vi "Read Current (List Voltage Sweep).vi"(5 "Delay Time (0.5 S)":dbl=0.5, 7 "Sweep Points (5)":i32=5, 8 "error in (no error)":errorcluster, 9 "Sweep List (V)":dbl[](array[numeric]), 10 "Source Measure Unit Channel (0: Channel A)":i32(ring) items=["Channel A", "Channel B"], 11 "VISA resource name":refnum<visa-resource-name>) -> (0 "error out":errorcluster, 2 "Current (A)":dbl[](array[numeric]), 3 "VISA resource name out":refnum<visa-resource-name>)   [LabVIEW 2015, in "Keithley 2600 Series.lvlib"]
doc: "Performs a voltage list sweep with current measured at every point."
uses:
  Keithley 2600 Series.lvlib
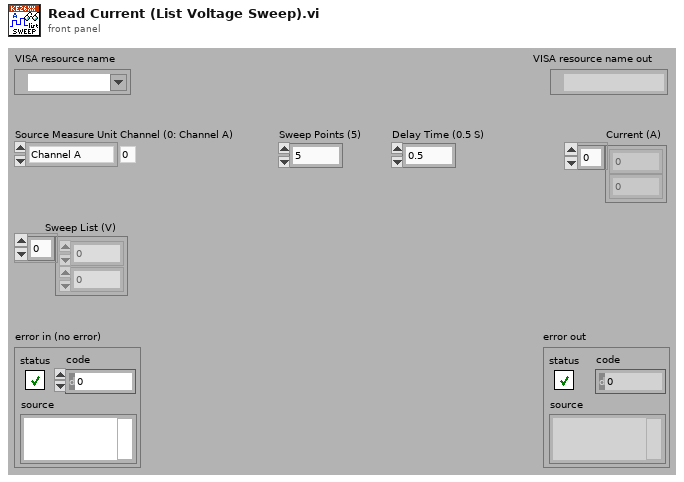
[diagram p1: front panel]
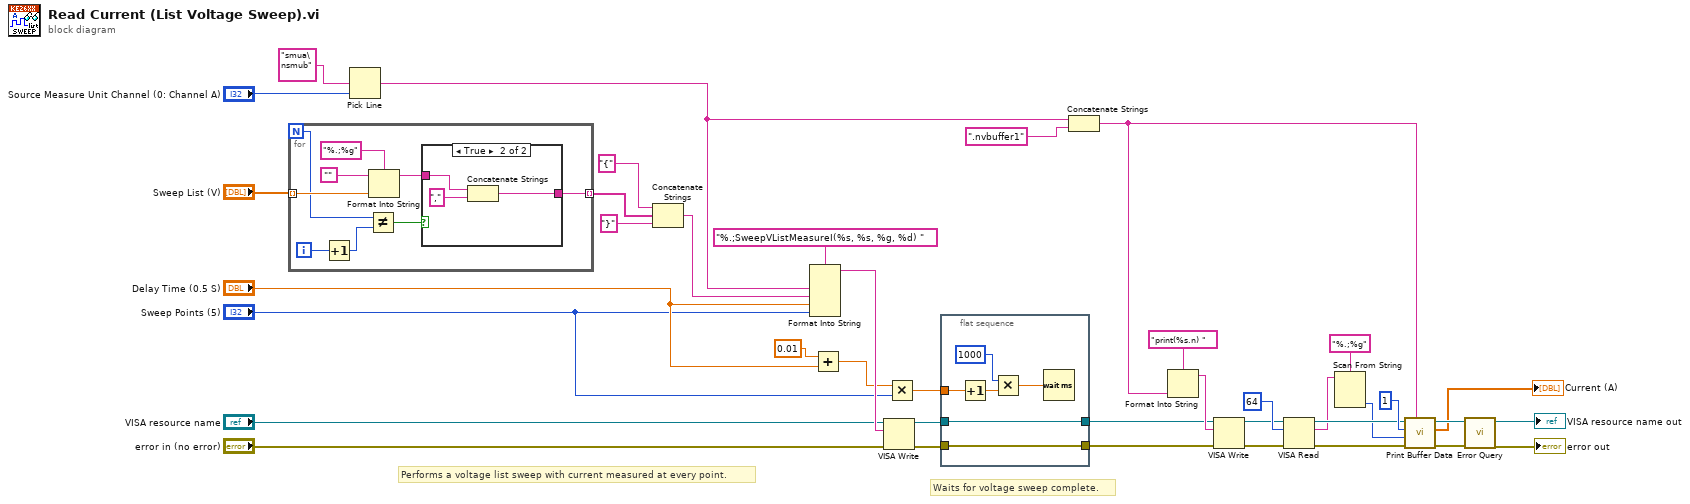
[diagram p0: block diagram]
diagram:
  # "Waits for voltage sweep complete."
  # "Performs a voltage list sweep with current measured at every point."
  n1 = for {
    N -> [w40]
    tunnel: "Sweep List (V)" -> [w48] mode=indexing
    tunnel: [w41] -> w31 mode=indexing
    i -> [w45]
    n2 = Increment(x=w45) -> (x+1=w44:i32)
    n3 = Not Equal?(x=w40, y=w44) -> (x != y?=w43:bool)
    n4 = Format Into String(format string="%.;%g", initial string="", w48) -> (resulting string=w42:string)  [unwired: 1 in, 1 out]
    n5 = case shown="True" w43 {
      tunnel: w42 -> [w49 w52]
      tunnel: [w49 w50] -> w41
      frame False {
      }
      frame True {
        n6 = Concatenate Strings(w52, ",") -> (w50:string)
      }
    }
  }
  n7 = Pick Line(multi-line string="smua\nsmub", line index="Source Measure Unit Channel (0: Channel A)") -> (output string=w6:string)  [unwired: 1 in]
  n8 = Concatenate Strings("{" ("string"), w31, "}") -> (w28:string)
  n9 = Format Into String(format string="%.;SweepVListMeasureI(%s, %s, %g, %d) ", w6, w28, "Delay Time (0.5 S)", "Sweep Points (5)") -> (resulting string=w38:string)  [unwired: 2 in, 1 out]
  n10 = Add(x=0.01, y="Delay Time (0.5 S)") -> (x+y=w22:dbl)
  n11 = VISA Write(VISA resource name="VISA resource name", write buffer=w38, error in (no error)="error in (no error)") -> (VISA resource name out=w26:refnum<visa-resource-name>, error out=w25:errorcluster)  [unwired: 1 out]
  n12 = Multiply(x=w22, y="Sweep Points (5)") -> (x*y=w20:dbl)
  n13 = flat-sequence {
    tunnel: w26 -> [w58]
    tunnel: w25 -> [w57]
    tunnel: [w58] -> w5
    tunnel: [w57] -> w4
    tunnel: w20 -> [w56]
    frame #0 {
      n14 = Increment(x=w56) -> (x+1=w55:dbl)
      n15 = Multiply(x=1000, y=w55) -> (x*y=w53:dbl)
      n16 = Wait (ms)(milliseconds to wait=w53) -> ()  [unwired: 1 out]
    }
  }
  n17 = Concatenate Strings(w6, ".nvbuffer1" ("string")) -> (w7:string)
  n18 = Format Into String(format string="print(%s.n) ", w7) -> (resulting string=w9:string)  [unwired: 2 in, 1 out]
  n19 = VISA Write(VISA resource name=w5, write buffer=w9, error in (no error)=w4) -> (VISA resource name out=w12:refnum<visa-resource-name>, error out=w11:errorcluster)  [unwired: 1 out]
  n20 = VISA Read(VISA resource name=w12, byte count=u32 64, error in (no error)=w11) -> (VISA resource name out=w17:refnum<visa-resource-name>, read buffer=w15:string, error out=w16:errorcluster)  [unwired: 1 out]
  n21 = Scan From String(format string="%.;%g", input string=w15) -> (output 1=w14:i32)  [unwired: 3 in, 3 out]
  n22 = call "Print Buffer Data.vi"("Reading Buffer (smua.nvbuffer1)"=w7, "error in (no error)"=w16, "End Index (1)"=w14, "Start Index (1)"=1 ("Start Index (0)"), "VISA resource name"=w17) -> ("error out"=w2:errorcluster, "Buffer Data"=→"Current (A)":dbl[], "VISA resource name out"=w3:refnum<visa-resource-name>)  [unwired: 4 in]
  n23 = call "Error Query.vi"("error in (no error)"=w2, "VISA resource name"=w3) -> ("error out"=→"error out":errorcluster, "VISA resource name out"=→"VISA resource name out":refnum<visa-resource-name>)  [unwired: 6 in, 2 out]
